vi "generateWaveform.vi"(8 "error in (no error)":errorcluster, 11 "IWaveform in":refnum<class "IWaveform.lvclass">) -> (0 "error out":errorcluster, 2 "Signal Out":dbl, 3 "IWaveform out":refnum<class "IWaveform.lvclass">)   [LabVIEW 2015, in "IWaveform.lvclass"]
uses:
  IWaveform.lvclass
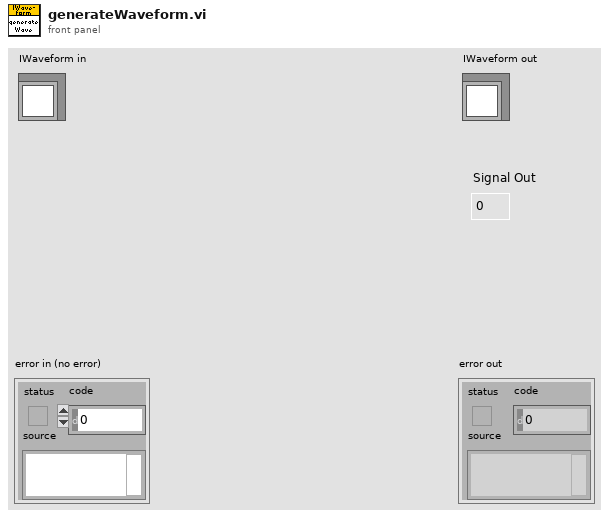
[diagram p1: front panel]
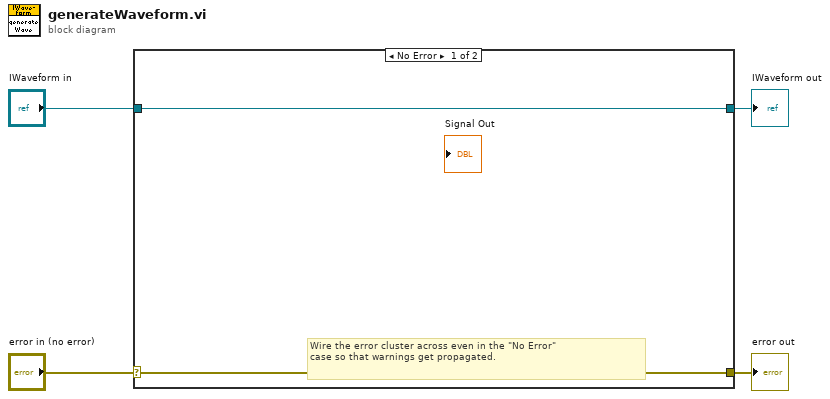
[diagram p0: block diagram]
diagram:
  n1 = case shown="No Error" "error in (no error)" {
    selector: "error in (no error)" -> [w5 w8]
    tunnel: [w5 w8] -> w3
    tunnel: [w6 w7] -> w1
    tunnel: "IWaveform in" -> [w6 w7]
    frame No Error {
      # "Wire the error cluster across even in the \"No Error\"\ncase so that warnings get propagated."
    }
    frame Error {
    }
  }
  "error out" <- w3
  "IWaveform out" <- w1
